vi "read maps dynamically.vi"(8 "error in":errorcluster, 11 "module configuration in":refnum<class "TBM module configuration.lvclass">) -> (0 "error out":errorcluster, 2 "maps dynamically":bool, 3 "module configuration out":refnum<class "TBM module configuration.lvclass">)   [LabVIEW 2013, in "TBM module configuration.lvclass"]
doc: "Provides an interface for determining if a runtime module associated with this configuration is capable of dynamically mapping to channels through <b>dynamic mapping.vi</b>."
uses:
  TBM module configuration.lvclass
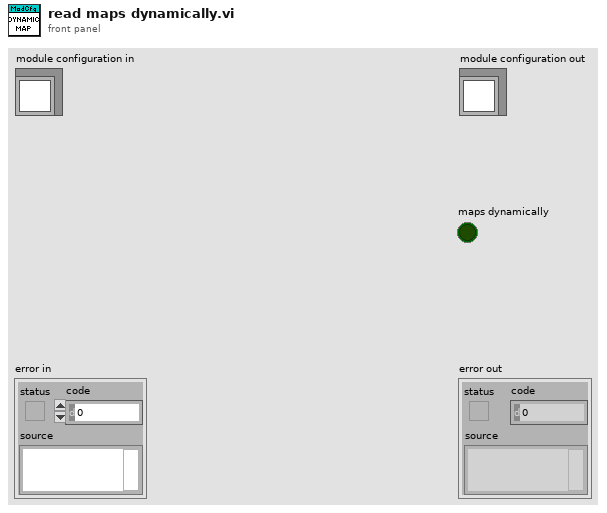
[diagram p1: front panel]
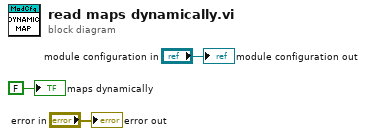
[diagram p0: block diagram]
diagram:
  "error out" <- "error in"
  "module configuration out" <- "module configuration in"
  "maps dynamically" <- FALSE ("maps dynamically")
